vi "Handle Messages.vi"(8 "error in (no error)":errorcluster, 9 "Message Data":variant, 10 "Message":string, 11 "Person In":refnum<class "Person.lvclass">) -> (0 "error out":errorcluster, 3 "Person Out":refnum<class "Person.lvclass">)   [LabVIEW 2020, in "Person.lvclass"]
uses:
  Person.lvclass
  C:/Program Files (x86)/National Instruments/LabVIEW 2020/vi.lib/Astemes/Triarc Framework/Process/Process.lvclass
  <vilib>/Astemes/Triarc Framework/Process/Process.lvclass/Process.ctl
  Person.lvclass/Person.ctl
  <vilib>/Astemes/Triarc Framework/Process/Protected/Messaging/Send Message.vi
  <vilib>/Astemes/Triarc Framework/Process/Private/SubVIs/Handle Debug Data.vi
  <vilib>/Astemes/Triarc Framework/Logging/Log Debug.vi
  <vilib>/AdvancedString/1D String Array to Delimited String.vi
  <vilib>/Utility/High Resolution Relative Seconds.vi
  <vilib>/Astemes/Triarc Framework/Process/Process.lvclass
  C:/Program Files (x86)/National Instruments/LabVIEW 2020/vi.lib/Astemes/Triarc Framework/Logging/Logging.lvclass
  <vilib>/Astemes/Triarc Framework/Process/Public/Lifecycle/Get Lifecycle State.vi
  <vilib>/Astemes/Triarc Framework/Process/Public/Read Name.vi
  <vilib>/Utility/error.llb/Error Cluster From Error Code.vi
  <vilib>/Astemes/Triarc Framework/Callback/Callback.lvclass
  <vilib>/Astemes/Triarc Framework/View/View.lvclass
  <vilib>/Astemes/Triarc Framework/Logging/Logging.lvclass
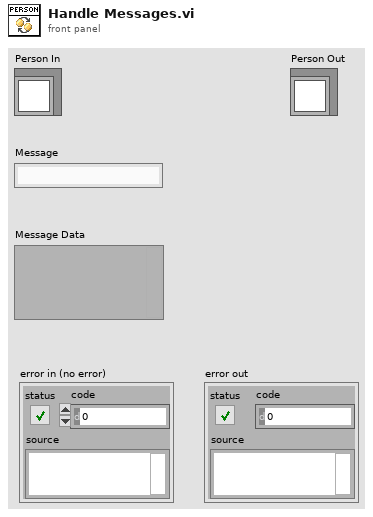
[diagram p1: front panel]
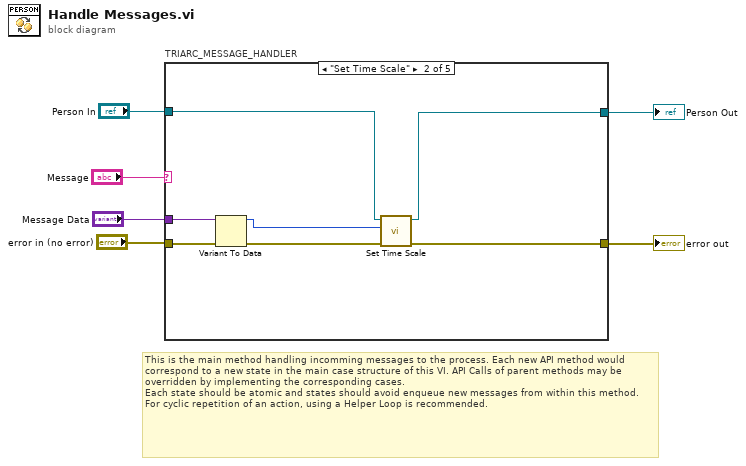
[diagram p0: block diagram]
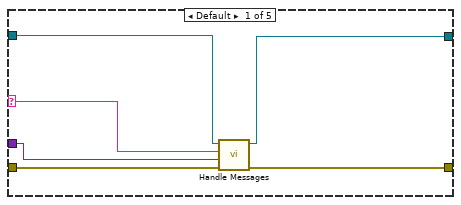
[diagram p2: hidden frame]
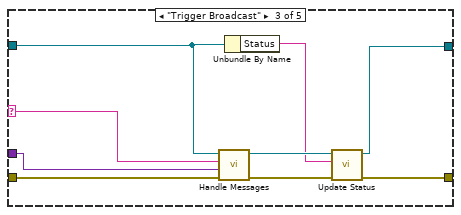
[diagram p3: hidden frame]
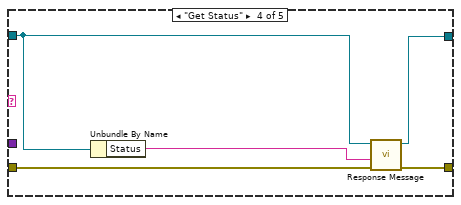
[diagram p4: hidden frame]
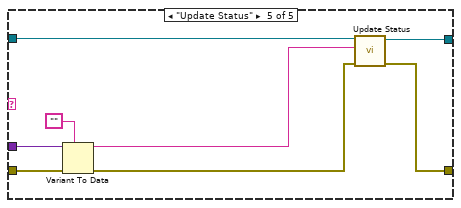
[diagram p5: hidden frame]
diagram:
  # "This is the main method handling incomming messages to the process. Each new API method would correspond to a new state in the main case structure of this VI. API Calls of parent methods may be overridden by implementing the corresponding cases.\nEach state should be atomic and states should avoid enqueue new messages from within this method. For cyclic repetition of an action, using a Helper Loop is recommended."
  n1 = case "TRIARC_MESSAGE_HANDLER" shown="\"Set Time Scale\"" "Message" {
    selector: "Message" -> [w10 _ w27 _ _]
    tunnel: "error in (no error)" -> [w9 w17 w26 w32 w37]
    tunnel: "Person In" -> [w12 w19 w21 w31 w34]
    tunnel: "Message Data" -> [w11 w18 w28 _ w40]
    tunnel: [w8 w13 w24 w29 w35] -> w2
    tunnel: [w7 w14 w22 w30 w36] -> w1
    frame Default {
      n2 = call-parent "Handle Messages.vi"("error in (no error)"=w9, "Message Data"=w11, "Message"=w10, "View In"=w12) -> ("error out"=w8:errorcluster, "View Out"=w7:refnum<class "Person.lvclass">)  [unwired: 6 in]
    }
    frame "Set Time Scale" {
      n3 = Variant To Data(error in=w17, Variant=w18) -> (data=w16:u32, error out=w15:errorcluster)  [unwired: 1 in]
      n4 = call "Set Time Scale.vi"("TRIARC_ERROR_IN"=w15, "Time Scale [ms]"=w16, "Person In"=w19) -> ("TRIARC_ERROR_OUT"=w13:errorcluster, "Person Out"=w14:refnum<class "Person.lvclass">)  [unwired: 7 in]
    }
    frame "Trigger Broadcast" {
      n5 = call-parent "Handle Messages.vi"("error in (no error)"=w26, "Message Data"=w28, "Message"=w27, "View In"=w21) -> ("error out"=w25:errorcluster, "View Out"=w23:refnum<class "Person.lvclass">)  [unwired: 6 in]
      n6 = Unbundle By Name(w21) -> ("Status"=w20:string)
      n7 = call "Update Status.vi"("error in (no error)"=w25, "Status"=w20, "Person In"=w23) -> ("error out"=w24:errorcluster, "Person Out"=w22:refnum<class "Person.lvclass">)  [unwired: 7 in]
    }
    frame "Get Status" {
      n8 = Unbundle By Name(w31) -> ("Status"=w33:string)
      n9 = call <vilib>:"Response Message.vi"("error in (no error)"=w32, "Response Message Data"=w33, "Process In"=w31) -> ("error out"=w29:errorcluster, "Process Out"=w30:refnum<class "Person.lvclass">)  [unwired: 7 in]
    }
    frame "Update Status" {
      n10 = Variant To Data(error in=w37, type="", Variant=w40) -> (data=w38:string, error out=w41:errorcluster)
      n11 = call "Update Status.vi"("error in (no error)"=w41, "Status"=w38, "Person In"=w34) -> ("error out"=w35:errorcluster, "Person Out"=w36:refnum<class "Person.lvclass">)  [unwired: 7 in]
    }
  }
  "error out" <- w2
  "Person Out" <- w1
